vi "PathPlanner_Waypoint_fromJSON.vi"(11 "JSON string":string) -> (0 "Error":bool, 3 "waypoints":T2[](array[typedef]) {"nextControl"."Y" format="%14.3f"; "nextControl"."X" format="%14.3f"; "anchor"."Y" format="%14.3f"; "anchor"."X" format="%14.3f"; "prevControl"."Y" format="%14.3f"; "prevControl"."X" format="%14.3f"}, 4 "value":T1(array[cluster]))   [LabVIEW 2019, in "PathPlanner24.lvlib"]
doc: "Create a waypoint from JSON text.\n\nInputs: \n - JSON String - string - JSON containing waypoint to parse and convert to waypoint\n\nOutputs:\n - Waypoints - array of waypoint - The waypoints created from JSON\n - error - boolean - TRUE if an error occured.\n - value - array of cluster - raw parse of JSON for debugging"
uses:
  PathPlanner24.lvlib
  TypeDef/PathPlannerWaypoint.ctl
  <vilib>/Rock Robotics/WPI/ThirdParty/JAS_Junk/TrajLib/TypeDef/TRANSLATION2D.ctl
  <vilib>/Rock Robotics/WPI/ThirdParty/JAS_Junk/TrajLib/Trajectory_Library.lvlib
panel:
  in  "waypoints":T1(array[cluster])
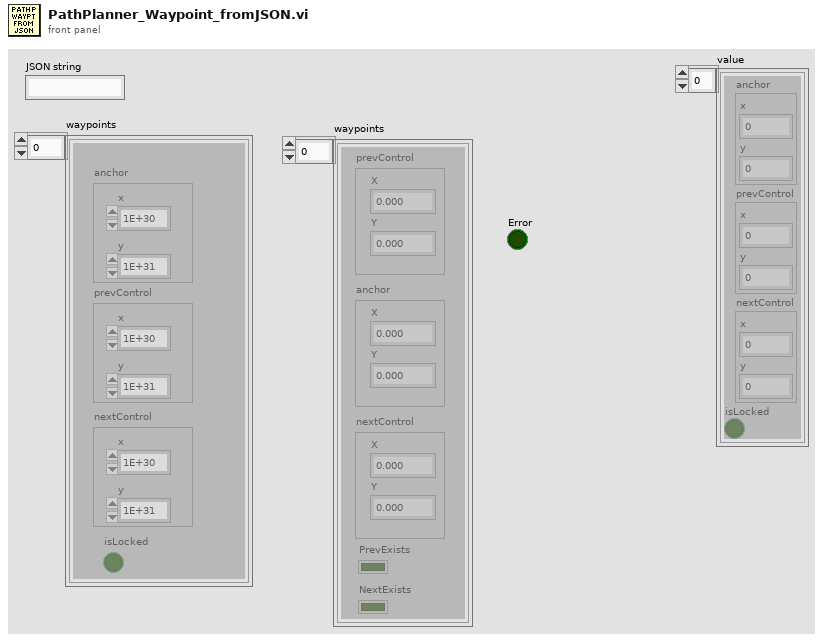
[diagram p1: front panel]
types:
  T1 = cluster{"anchor":cluster{"x":dbl, "y":dbl}, "prevControl":cluster{"x":dbl, "y":dbl}, "nextControl":cluster{"x":dbl, "y":dbl}, "isLocked":bool}[]
  T2 = typedef "PathPlanner24.lvlib/PathPlannerWaypoint.ctl" = cluster{"prevControl":T3, "anchor":T3, "nextControl":T3, "PrevExists":bool, "NextExists":bool}
  T3 = typedef "Trajectory_Library.lvlib/TRANSLATION2D.ctl" = cluster{"X":dbl, "Y":dbl}
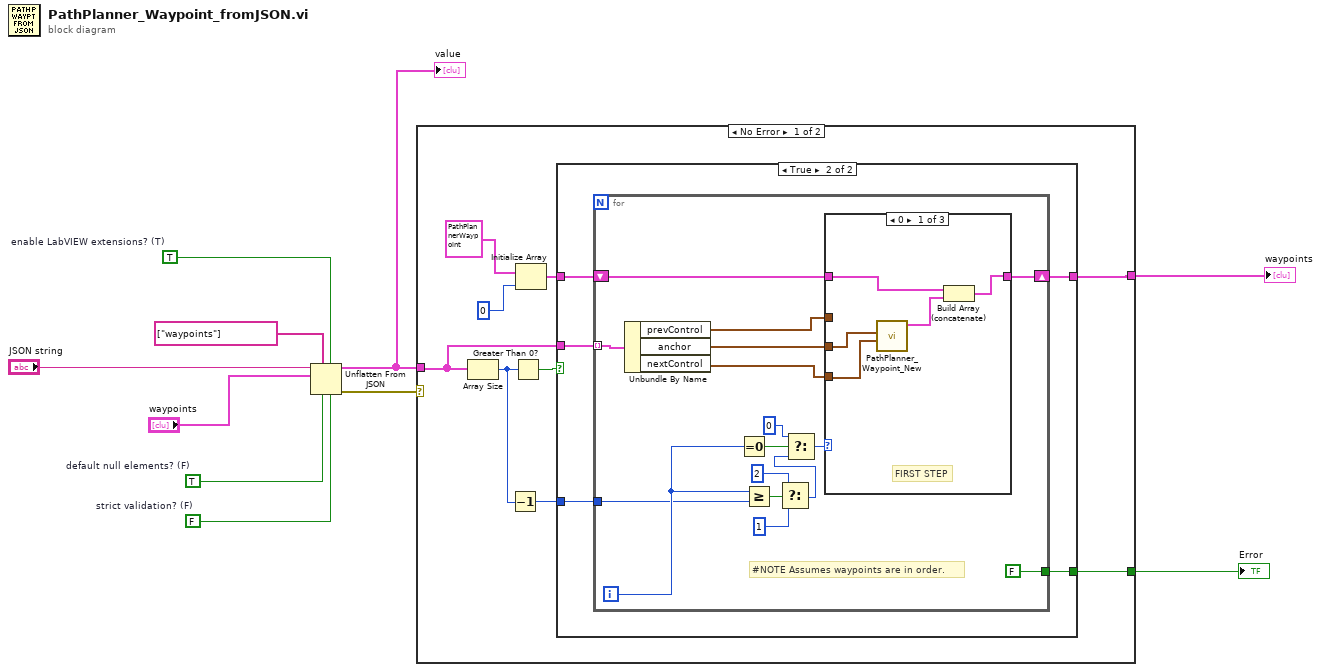
[diagram p0: block diagram]
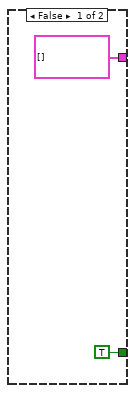
[diagram p2: hidden frame]
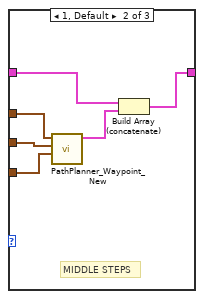
[diagram p3: hidden frame]
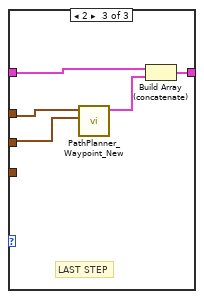
[diagram p4: hidden frame]
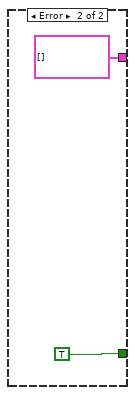
[diagram p5: hidden frame]
diagram:
  w5 = TRUE  # default null elements? (F)
  w6 = FALSE  # strict validation? (F)
  w7 = TRUE  # enable LabVIEW extensions? (T)
  n1 = Unflatten From JSON(path=string[] ["waypoints"], enable LabVIEW extensions? (T)=w7, JSON string="JSON string", type and defaults="waypoints", default null elements? (F)=w5, strict validation? (F)=w6) -> (value=w2:T1, error out=w8:errorcluster)  [unwired: 1 in]
  "value" <- w2
  n2 = case shown="No Error" w8 {
    tunnel: w2 -> [w13 _]
    tunnel: [w11 TRUE] -> w3
    tunnel: [w12 T2[] []] -> w1
    frame No Error {
      n3 = Array Size(array=w13) -> (size(s)=w18:i32)
      n4 = Decrement(x=w18) -> (x-1=w17:i32)
      n5 = Greater Than 0?(x=w18) -> (x > 0?=w19:bool)
      n6 = Initialize Array(T2 {"prevControl"={"X"=0.0, "Y"=0.0}, "anchor"={"X"=0.0, "Y"=0.0}, "nextControl"={"X"=0.0, "Y"=0.0}, "PrevExists"=FALSE, "NextExists"=FALSE} ("Bezier"), 0 ("dimension size")) -> (w14:T2[])
      n7 = case shown="True" w19 {
        tunnel: w17 -> [_ w26]
        tunnel: w14 -> [_ w25]
        tunnel: w13 -> [_ w24]
        tunnel: [T2[] [] w23] -> w12
        tunnel: [TRUE w22] -> w11
        frame False {
        }
        frame True {
          n8 = for {
            tunnel: w26 -> [w27]
            shift-right: [w31] -> w23
            shift-left: w25 -> [w36]
            tunnel: w24 -> [w37] mode=indexing
            tunnel: [FALSE] -> w22
            i -> [w28]
            # "#NOTE Assumes waypoints are in order."
            n9 = Unbundle By Name(w37) -> ("prevControl"=w35:cluster{"x":dbl, "y":dbl}, "anchor"=w34:cluster{"x":dbl, "y":dbl}, "nextControl"=w33:cluster{"x":dbl, "y":dbl})
            n10 = Equal To 0?(x=w28) -> (x = 0?=w30:bool)
            n11 = Greater Or Equal?(x=w28, y=w27) -> (x >= y?=w29:bool)
            n12 = Select(t=2, s=w29, f=1) -> (s? t:f=w39:i32)
            n13 = Select(t=0, s=w30, f=w39) -> (s? t:f=w38:i32)
            n14 = case shown="0" w38 {
              tunnel: w36 -> [w44 w49 w56]
              tunnel: w35 -> [_ w52 w58]
              tunnel: w34 -> [w46 w51 w57]
              tunnel: w33 -> [w45 w50 _]
              tunnel: [w43 w48 w54] -> w31
              frame 0 {
                # "FIRST STEP"
                n15 = call "PathPlanner_Waypoint_New.vi"("NextControl"=w45, "Anchor"=w46) -> ("Waypoint"=w47:T2)  [unwired: 9 in]
                n16 = Build Array (concatenate)(w44, w47) -> (w43:T2[])
              }
              frame 1, Default {
                # "MIDDLE STEPS"
                n17 = call "PathPlanner_Waypoint_New.vi"("NextControl"=w50, "Anchor"=w51, "PrevControl"=w52) -> ("Waypoint"=w53:T2)  [unwired: 8 in]
                n18 = Build Array (concatenate)(w49, w53) -> (w48:T2[])
              }
              frame 2 {
                # "LAST STEP"
                n19 = call "PathPlanner_Waypoint_New.vi"("Anchor"=w57, "PrevControl"=w58) -> ("Waypoint"=w55:T2)  [unwired: 9 in]
                n20 = Build Array (concatenate)(w56, w55) -> (w54:T2[])
              }
            }
          }
        }
      }
    }
    frame Error {
    }
  }
  "waypoints" <- w1
  "Error" <- w3
